vi "9230_DAQmx (subVI).vi"(0 "DAQ Device":tag="cDAQ1Mod1", 1 "ai0_sensitivity":dbl=14.0320637122449 format="%#_15g", 2 "ai1_sensitivity":dbl=13.8991380183673 format="%#_15g", 3 "ai2_sensitivity":dbl=14.0350854918367 format="%#_15g", 5 "number of samples":i32=10000, 7 "rate":dbl=10000.0 format="%0.2f", 11 "error in":errorcluster) -> (4 "task out":refnum<k21>, 15 "error out":errorcluster)   [LabVIEW 2018]
uses:
  <vilib>/DAQmx/create/channels.llb/DAQmx Create Channel (AI-Acceleration-Accelerometer).vi
  <vilib>/DAQmx/configure/timing.llb/DAQmx Timing (Sample Clock).vi
  <resource>/objmgr/daqmx.rc
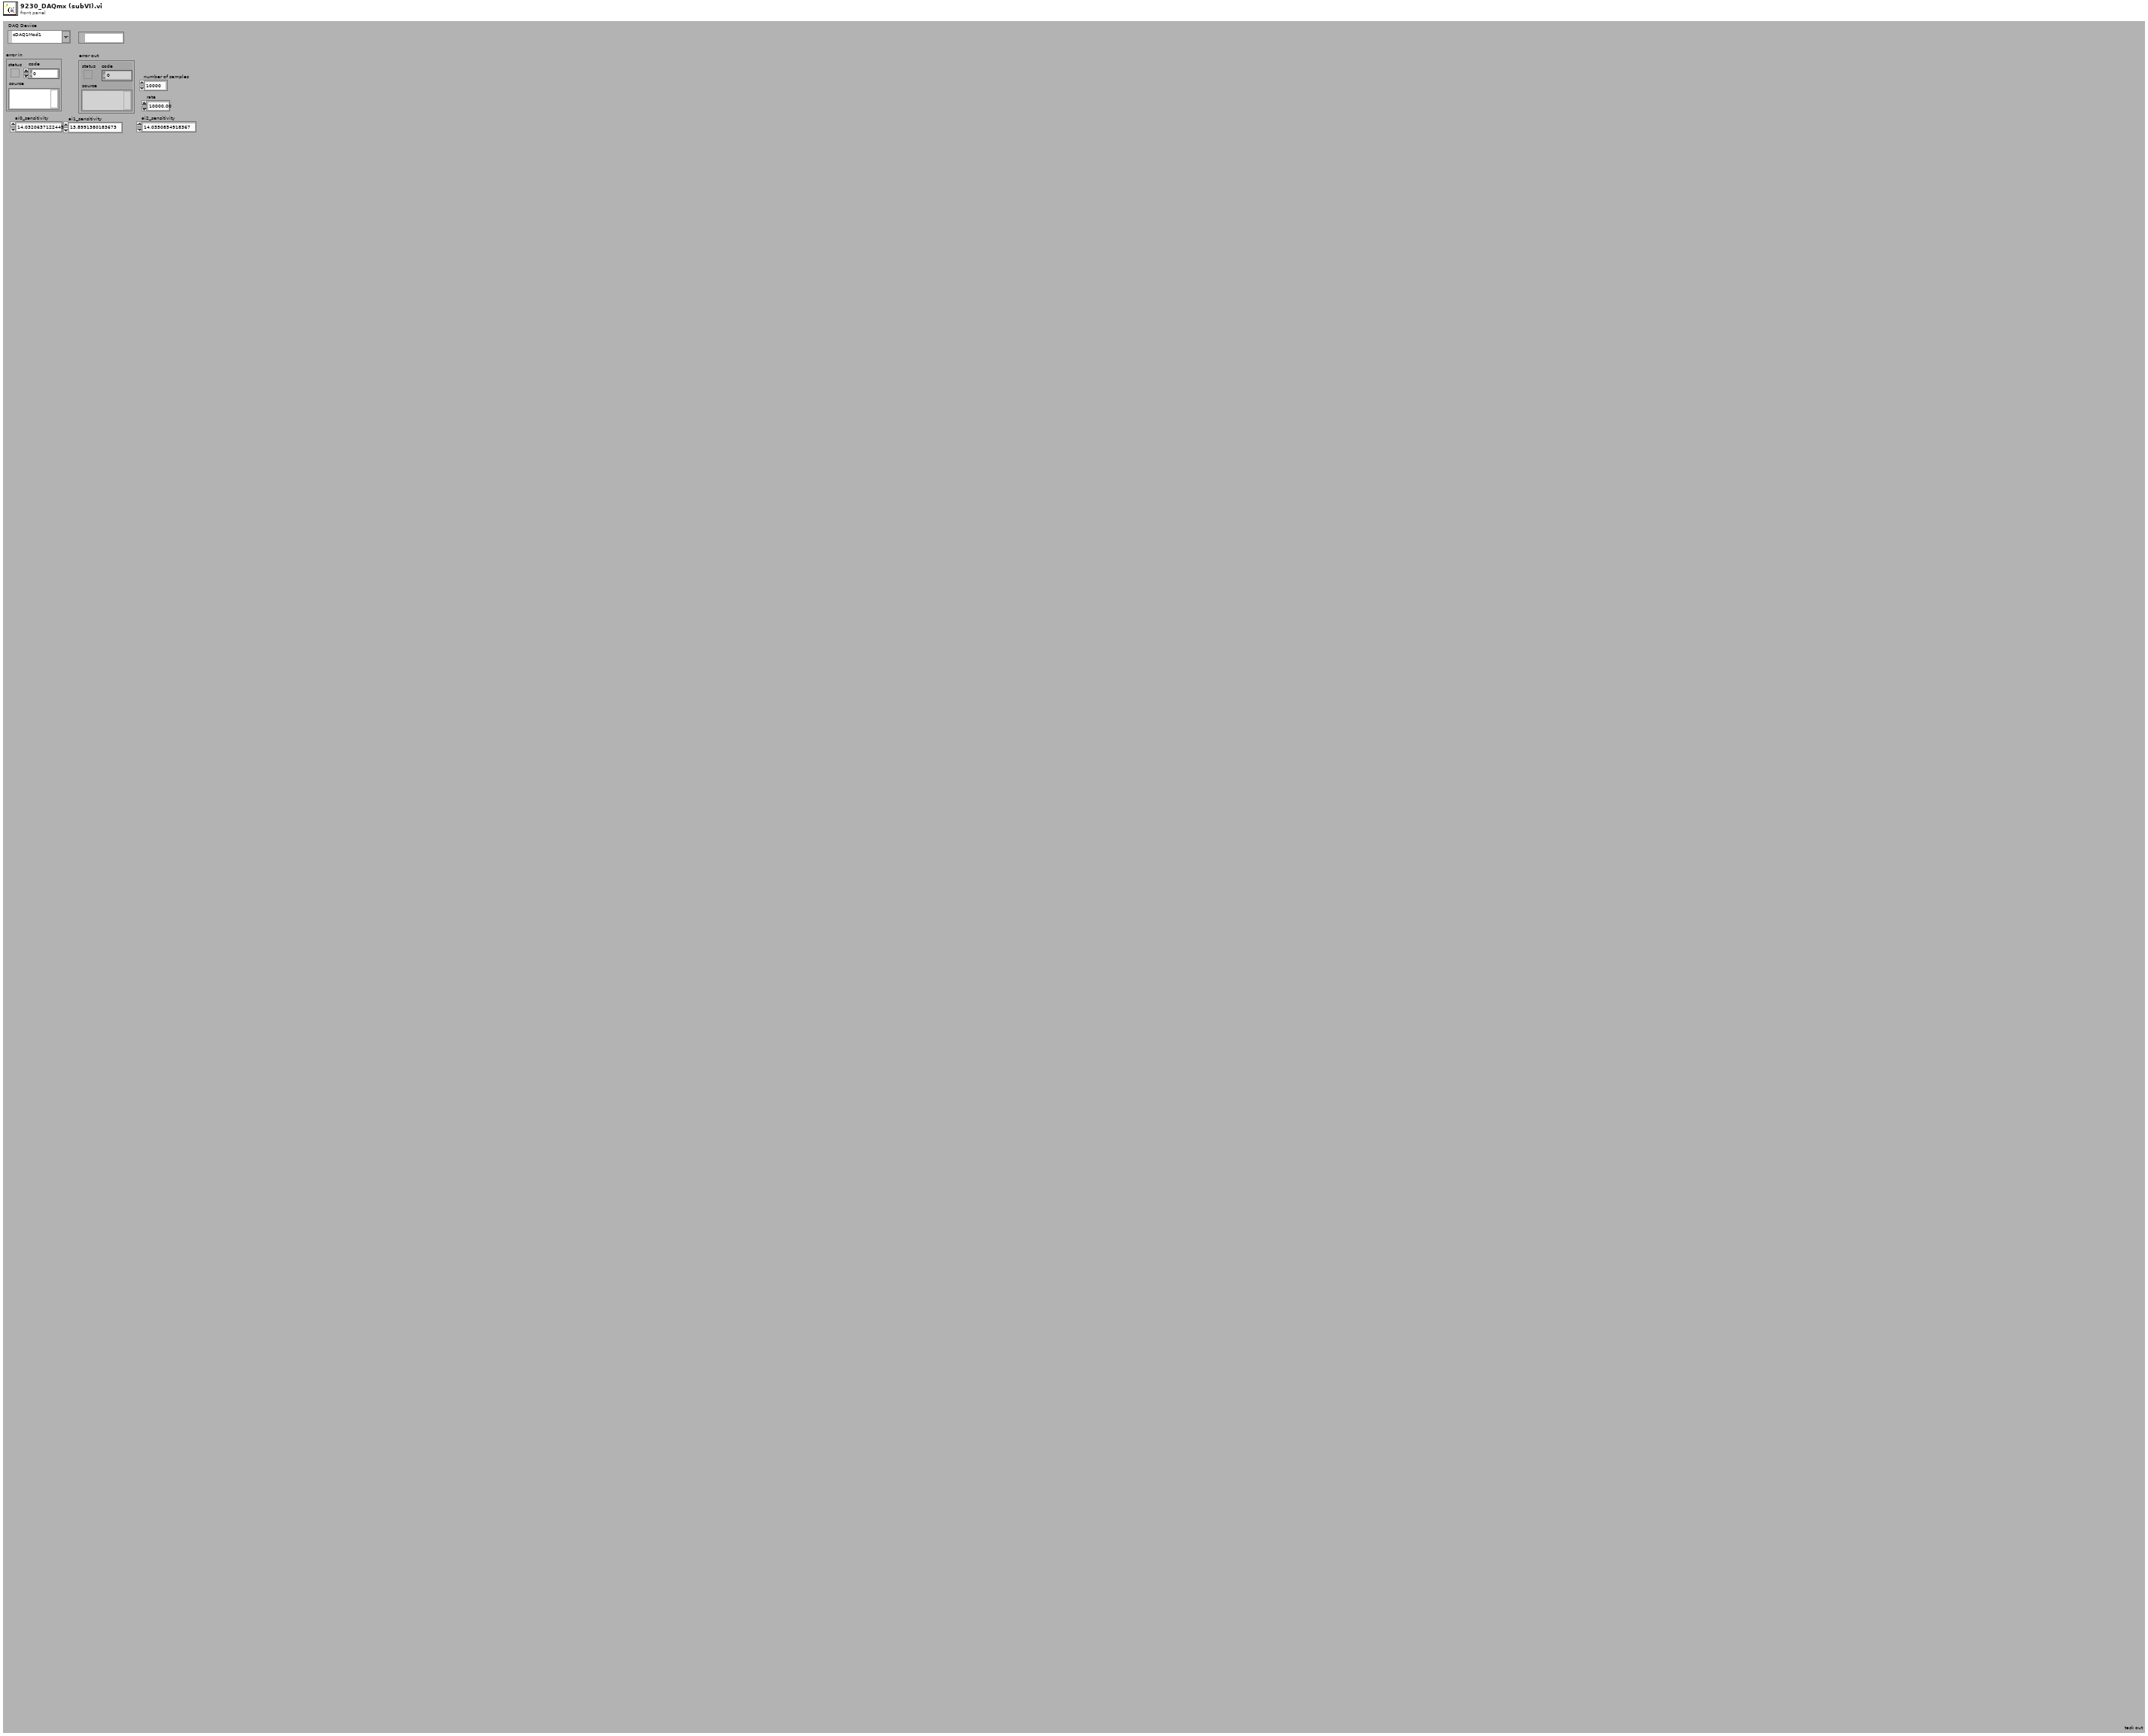
[diagram p1: front panel]
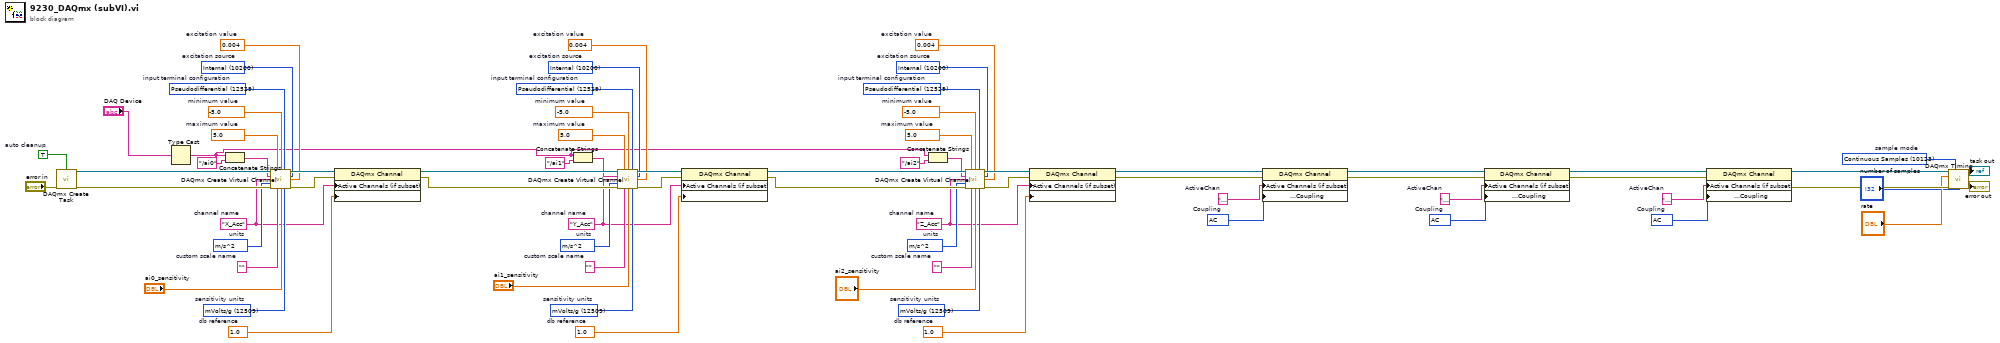
[diagram p0: block diagram]
diagram:
  w9 = 10123 items=["Finite Samples"=10178, "Continuous Samples"=10123, "Hardware Timed Single Point"=12522]  # sample mode
  w17 = 10045 items=["AC"=10045, "DC"=10050, "GND"=10066]  # Coupling
  w18 = "Z_Acc"  # ActiveChan
  w21 = 10045 items=["AC"=10045, "DC"=10050, "GND"=10066]  # Coupling
  w22 = "Y_Acc"  # ActiveChan
  w25 = 10045 items=["AC"=10045, "DC"=10050, "GND"=10066]  # Coupling
  w26 = "X_Acc"  # ActiveChan
  w28 = 1.0  # db reference
  w31 = 12470 items=["g"=10186, "m/s^2"=12470, "From Custom Scale"=10065]  # units
  w32 = 12529 items=["default"=-1, "RSE"=10083, "NRSE"=10078, "Differential"=10106, "Pseudodifferential"=12529]  # input terminal configuration
  w33 = 10200 items=["Internal"=10200, "External"=10167, "None"=10230]  # excitation source
  w34 = 0.004  # excitation value
  w35 = 12509 items=["mVolts/g"=12509, "Volts/g"=12510]  # sensitivity units
  w27 = "Z_Acc"  # channel name
  w38 = ""  # custom scale name
  w39 = -5.0  # minimum value
  w40 = 5.0  # maximum value
  w43 = 1.0  # db reference
  w46 = 12470 items=["g"=10186, "m/s^2"=12470, "From Custom Scale"=10065]  # units
  w47 = 12529 items=["default"=-1, "RSE"=10083, "NRSE"=10078, "Differential"=10106, "Pseudodifferential"=12529]  # input terminal configuration
  w48 = 10200 items=["Internal"=10200, "External"=10167, "None"=10230]  # excitation source
  w49 = 0.004  # excitation value
  w50 = 12509 items=["mVolts/g"=12509, "Volts/g"=12510]  # sensitivity units
  w42 = "Y_Acc"  # channel name
  w53 = ""  # custom scale name
  w54 = -5.0  # minimum value
  w55 = 5.0  # maximum value
  w58 = 1.0  # db reference
  w61 = 12470 items=["g"=10186, "m/s^2"=12470, "From Custom Scale"=10065]  # units
  w62 = 12529 items=["default"=-1, "RSE"=10083, "NRSE"=10078, "Differential"=10106, "Pseudodifferential"=12529]  # input terminal configuration
  w63 = 10200 items=["Internal"=10200, "External"=10167, "None"=10230]  # excitation source
  w64 = 0.004  # excitation value
  w65 = 12509 items=["mVolts/g"=12509, "Volts/g"=12510]  # sensitivity units
  w57 = "X_Acc"  # channel name
  w68 = ""  # custom scale name
  w69 = -5.0  # minimum value
  w70 = 5.0  # maximum value
  w72 = TRUE  # auto cleanup
  n1 = call <vilib>:"DAQmx Create Task.vi"("auto cleanup"=w72, "error in"="error in") -> ("task out"=w71:refnum<k21>, "error out"=w73:errorcluster)  [unwired: 12 in]
  n2 = Type Cast(x="DAQ Device") -> (*(type *) &x=w2:string)  [unwired: 1 in]
  n3 = Concatenate Strings(w2, "/ai0" ("string")) -> (w7:string)
  n4 = call-poly <vilib>:"DAQmx Create Virtual Channel.vi"("task in"=w71, "maximum value"=w70, "minimum value"=w69, "input terminal configuration"=w62, "physical channels"=w7, "current excitation source"=w63, "name to assign"=w57, "current excitation value"=w64, "units"=w61, "error in"=w73, "custom scale name"=w68, "sensitivity"="ai0_sensitivity", "sensitivity units"=w65) -> ("task out"=w67:refnum<k21>, "error out"=w60:errorcluster)  [unwired: 1 in]
  n5 = property class="DAQmx Channel"(reference=w67, error in=w60, "Active Channels (if subset)"=w57, "Analog Input:Acceleration:dB Reference"=w58) -> (reference out=w56:refnum<k21>, error out=w59:errorcluster)
  n6 = Concatenate Strings(w2, "/ai1" ("string")) -> (w5:string)
  n7 = call-poly <vilib>:"DAQmx Create Virtual Channel.vi"("task in"=w56, "maximum value"=w55, "minimum value"=w54, "input terminal configuration"=w47, "physical channels"=w5, "current excitation source"=w48, "name to assign"=w42, "current excitation value"=w49, "units"=w46, "error in"=w59, "custom scale name"=w53, "sensitivity"="ai1_sensitivity", "sensitivity units"=w50) -> ("task out"=w52:refnum<k21>, "error out"=w45:errorcluster)  [unwired: 1 in]
  n8 = property class="DAQmx Channel"(reference=w52, error in=w45, "Active Channels (if subset)"=w42, "Analog Input:Acceleration:dB Reference"=w43) -> (reference out=w41:refnum<k21>, error out=w44:errorcluster)
  n9 = Concatenate Strings(w2, "/ai2" ("string")) -> (w3:string)
  n10 = call-poly <vilib>:"DAQmx Create Virtual Channel.vi"("task in"=w41, "maximum value"=w40, "minimum value"=w39, "input terminal configuration"=w32, "physical channels"=w3, "current excitation source"=w33, "name to assign"=w27, "current excitation value"=w34, "units"=w31, "error in"=w44, "custom scale name"=w38, "sensitivity"="ai2_sensitivity", "sensitivity units"=w35) -> ("task out"=w37:refnum<k21>, "error out"=w30:errorcluster)  [unwired: 1 in]
  n11 = property class="DAQmx Channel"(reference=w37, error in=w30, "Active Channels (if subset)"=w27, "Analog Input:Acceleration:dB Reference"=w28) -> (reference out=w23:refnum<k21>, error out=w29:errorcluster)
  n12 = property class="DAQmx Channel"(reference=w23, error in=w29, "Active Channels (if subset)"=w26, "Analog Input:General Properties:Input Configuration:Coupling"=w25) -> (reference out=w19:refnum<k21>, error out=w24:errorcluster)
  n13 = property class="DAQmx Channel"(reference=w19, error in=w24, "Active Channels (if subset)"=w22, "Analog Input:General Properties:Input Configuration:Coupling"=w21) -> (reference out=w15:refnum<k21>, error out=w20:errorcluster)
  n14 = property class="DAQmx Channel"(reference=w15, error in=w20, "Active Channels (if subset)"=w18, "Analog Input:General Properties:Input Configuration:Coupling"=w17) -> (reference out=w12:refnum<k21>, error out=w16:errorcluster)
  n15 = call-poly <vilib>:"DAQmx Timing.vi"("task/channels in"=w12, "sample mode"=w9, "samples per channel"="number of samples", "rate"="rate", "error in"=w16) -> ("task out"=→"task out":refnum<k21>, "error out"=→"error out":errorcluster)  [unwired: 9 in]
